vi "View.vi"(8 "error in (no error)":errorcluster, 11 "Thermal Chamber Controller In":refnum<class "Thermal Chamber Controller.lvclass">) -> (0 "error out":errorcluster)   [LabVIEW 2020, in "Thermal Chamber Controller.lvclass"]
doc: "This VI implements the main UI of the process. A reference to this VI should be set using the Set View VI Reference.vi method when the VI is started."
uses:
  Thermal Chamber Controller.lvclass
  C:/Program Files (x86)/National Instruments/LabVIEW 2020/vi.lib/Astemes/Triarc Framework/Process/Process.lvclass
  C:/Program Files (x86)/National Instruments/LabVIEW 2020/vi.lib/Astemes/Triarc Framework/View/View.lvclass
  <vilib>/Astemes/Triarc Framework/View/View.lvclass/View.ctl
  Thermal Chamber Controller.lvclass/Thermal Chamber Controller.ctl
  Private/Heater State.ctl
  <vilib>/Astemes/Triarc Framework/View/View.lvclass
  <vilib>/Astemes/Triarc Framework/Process/Process.lvclass
  C:/Program Files (x86)/National Instruments/LabVIEW 2020/vi.lib/Asteme/Triarc Framework/View/View.lvclass
  C:/Program Files (x86)/National Instruments/LabVIEW 2020/vi.lib/Asteme/Triarc Framework/Process/Process.lvclass
  C:/Program Files (x86)/National Instruments/LabVIEW 2020/vi.lib/Asteme/Triarc Framework/Base/Base.lvclass
  C:/Program Files (x86)/National Instruments/LabVIEW 2020/vi.lib/Asteme/Triarc Framework/Error Handler Interface/Error Handler Interface.lvclass
  C:/Program Files (x86)/National Instruments/LabVIEW 2020/vi.lib/Asteme/Triarc Framework/Logging/Logging.lvclass
  C:/Users/anton/Documents/GitHub/Triarc-Examples/Thermal Chamber/Thermal Chamber Controller/Thermal Chamber Controller.lvclass
  C:/Program Files (x86)/National Instruments/LabVIEW 2020/vi.lib/Asteme/Triarc Framework/Helper Loop/Helper Loop.lvclass
panel:
  in  "Enable Heater":bool
  in  "Disable Heater":bool
  in  "Ramp Rate (deg C / second)":dbl=1.0
  in  "Temperature Set Point (deg C)":dbl=22.0
  out "Heater State":bool
  out "Actual Temperature":dbl format="%.2f"
  out "Chamber Temperature Chart":T1(graph)
  out "Status":string
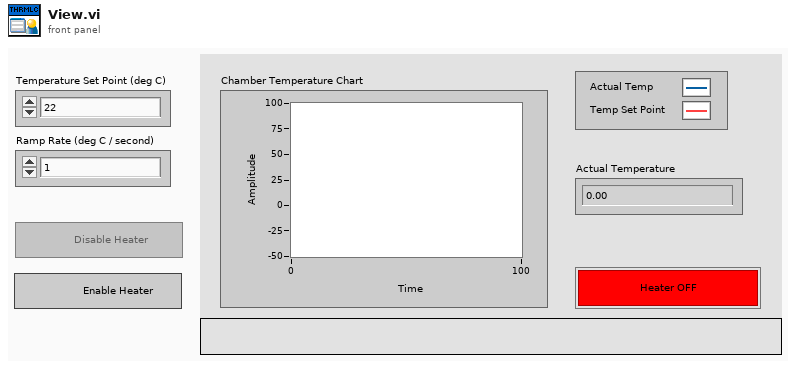
[diagram p1: front panel]
types:
  T1 = cluster{"Actual Temperature":dbl, "Required Temperature deg C":dbl}
  T2 = cluster{"Actual Temperature":dbl, "Required Temperature deg C":dbl}[]
  T3 = typedef "Thermal Chamber Controller.lvclass/Heater State.ctl" = enum16{"Heater Disabled", "Heater Enabled"}
  T4 = cluster{"Actual Temperature":dbl, "Temperature Set Point":dbl}
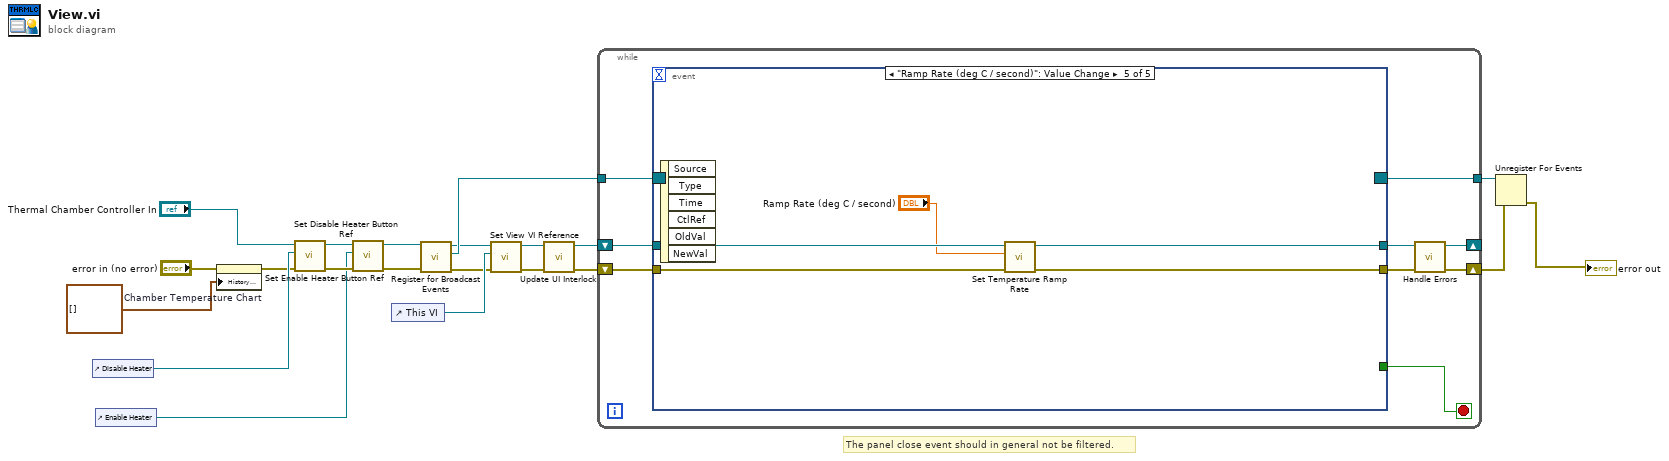
[diagram p0: block diagram]
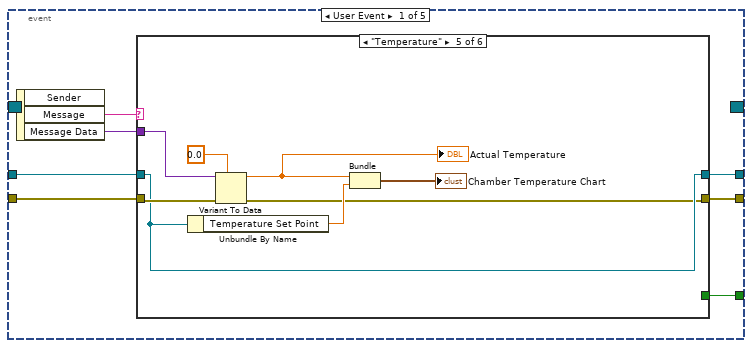
[diagram p2: hidden frame]
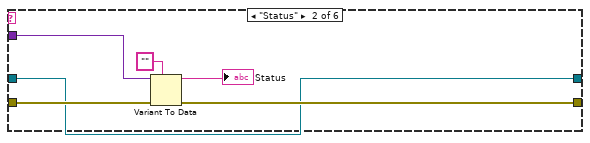
[diagram p4: hidden frame]
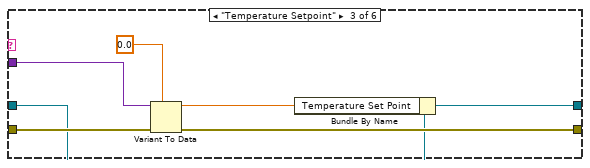
[diagram p5: hidden frame]
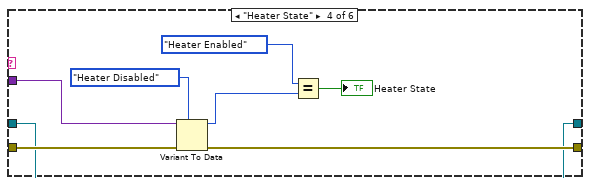
[diagram p6: hidden frame]
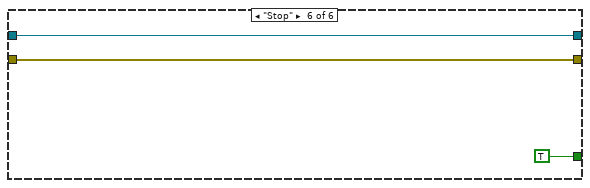
[diagram p7: hidden frame]
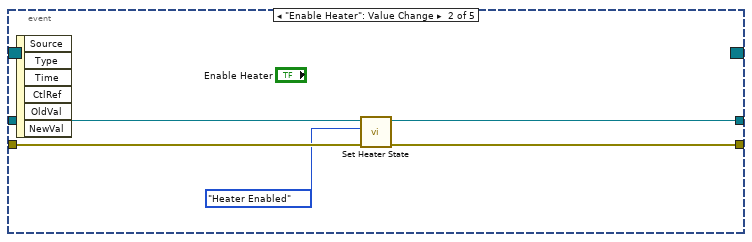
[diagram p8: hidden frame]
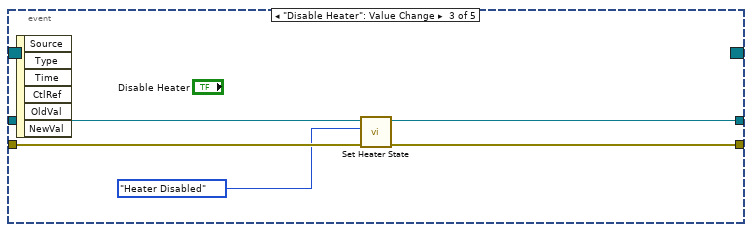
[diagram p9: hidden frame]
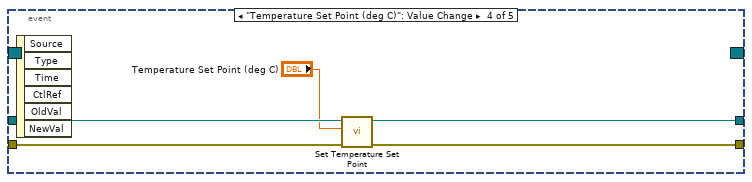
[diagram p10: hidden frame]
diagram:
  # "The panel close event should in general not be filtered."
  n1 = control-ref of="Disable Heater"() -> (w8:refnum<vi>)
  n2 = control-ref of="Enable Heater"() -> (w7:refnum<vi>)
  n3 = property on="Chamber Temperature Chart" class="WFChart (strict)"(error in="error in (no error)", "History Data"=T2 []) -> (error out=w2:errorcluster)  [unwired: 1 in, 1 out]
  n4 = call "Set Disable Heater Button Ref.vi"("error in (no error)"=w2, "Disable Heater Button Ref"=w8, "Thermal Chamber Controller In"="Thermal Chamber Controller In") -> ("error out"=w11:errorcluster, "Thermal Chamber Controller Out"=w9:refnum<class "Thermal Chamber Controller.lvclass">)  [unwired: 7 in]
  n5 = call "Set Enable Heater Button Ref.vi"("error in (no error)"=w11, "Enable Heater Button Ref"=w7, "Thermal Chamber Controller In"=w9) -> ("error out"=w13:errorcluster, "Thermal Chamber Controller Out"=w12:refnum<class "Thermal Chamber Controller.lvclass">)  [unwired: 7 in]
  n6 = control-ref of="This VI"() -> (w20:refnum<vi>)
  n7 = call <vilib>:"Register for Broadcast Events.vi"("error in (no error)"=w13, "Process In"=w12) -> ("error out"=w18:errorcluster, "Event Registration Refnum Out"=w19:refnum<event-registration>, "Process Out"=w17:refnum<class "Thermal Chamber Controller.lvclass">)  [unwired: 7 in]
  n8 = call <vilib>:"Set View VI Reference.vi"("error in (no error)"=w18, "View VI Reference"=w20, "View In"=w17) -> ("error out"=w16:errorcluster, "View Out"=w5:refnum<class "Thermal Chamber Controller.lvclass">)  [unwired: 7 in]
  n9 = call "Update UI Interlock.vi"("error in (no error)"=w16, "Thermal Chamber Controller In"=w5) -> ("error out"=w6:errorcluster, "Thermal Chamber Controller Out"=w4:refnum<class "Thermal Chamber Controller.lvclass">)  [unwired: 8 in]
  n10 = while {
    shift-right: [w24] -> _
    shift-left: w4 -> [w30]
    shift-right: [w22] -> w15
    shift-left: w6 -> [w28]
    tunnel: w19 -> [w27]
    tunnel: [w26] -> w14
    stop <- w25 stop-if-true
    n11 = event shown="[4] \"Ramp Rate (deg C / second)\": Value Change" {
      selector: w27 -> [_ _ _ _ _]
      dyn-events: [_ _ _ _ _] -> w26
      timeout: _ -> [_ _ _ _ _]
      tunnel: w30 -> [w37 w74 w79 w86 w89]
      tunnel: [w36 w73 w78 w85 w88] -> w29
      tunnel: w28 -> [w34 w76 w81 w83 w91]
      tunnel: [w35 w75 w80 w84 w90] -> w23
      tunnel: [w32 _ _ _ _] -> w25
      event User Event {
        n12 = event-data() -> ("Message"=w33:string, "Message Data"=w31:variant)  [unwired: 1 in, 1 out]
        n13 = case shown="\"Temperature\"" w33 {
          tunnel: w37 -> [w39 w40 w49 w53 w63 w71]
          tunnel: [w39 w40 w47 w53 w63 w71] -> w36
          tunnel: [w38 w41 w50 w57 w62 w70] -> w35
          tunnel: w34 -> [w38 w44 w51 w58 w68 w70]
          tunnel: [_ _ _ _ _ TRUE] -> w32
          tunnel: w31 -> [_ w45 w52 w59 w67 _]
          frame Default {
          }
          frame "Status" {
            n14 = Variant To Data(error in=w44, type="", Variant=w45) -> (data=→"Status":string, error out=w41:errorcluster)
          }
          frame "Temperature Setpoint" {
            n15 = Variant To Data(error in=w51, type=0.0 ("Numeric"), Variant=w52) -> (data=w46:dbl, error out=w50:errorcluster)
            n16 = Bundle By Name(cluster=w49, "Temperature Set Point"=w46) -> (w47:refnum<class "Thermal Chamber Controller.lvclass">)
          }
          frame "Heater State" {
            n17 = Variant To Data(error in=w58, type=Heater_State."Heater Disabled" ("Heater State"), Variant=w59) -> (data=w55:T3, error out=w57:errorcluster)
            n18 = Equal?(x=Heater_State."Heater Enabled" ("Heater State"), y=w55) -> (x = y?=→"Heater State":bool)
          }
          frame "Temperature" {
            n19 = Unbundle By Name(w63) -> ("Temperature Set Point"=w64:dbl)
            n20 = Variant To Data(error in=w68, type=0.0 ("Actual Temperature"), Variant=w67) -> (data=w65:dbl, error out=w62:errorcluster)
            "Actual Temperature" <- w65
            n21 = Bundle("Actual Temperature"=w65, "Temperature Set Point"=w64) -> (→"Chamber Temperature Chart":T4)  [unwired: 1 in]
          }
          frame "Stop" {
          }
        }
      }
      event "Enable Heater": Value Change {
        n22 = event-data() -> ()  [unwired: 1 in, 6 out]
        n23 = call "Set Heater State.vi"("error in (no error)"=w76, "Heater State"=Heater_State."Heater Enabled", "Thermal Chamber Controller In"=w74) -> ("error out"=w75:errorcluster, "Thermal Chamber Controller Out"=w73:refnum<class "Thermal Chamber Controller.lvclass">)  [unwired: 7 in]
      }
      event "Disable Heater": Value Change {
        n24 = event-data() -> ()  [unwired: 1 in, 6 out]
        n25 = call "Set Heater State.vi"("error in (no error)"=w81, "Heater State"=Heater_State."Heater Disabled", "Thermal Chamber Controller In"=w79) -> ("error out"=w80:errorcluster, "Thermal Chamber Controller Out"=w78:refnum<class "Thermal Chamber Controller.lvclass">)  [unwired: 7 in]
      }
      event "Temperature Set Point (deg C)": Value Change {
        n26 = event-data() -> ()  [unwired: 1 in, 6 out]
        n27 = call "Set Temperature Set Point.vi"("error in (no error)"=w83, "Temperature Set Point"="Temperature Set Point (deg C)", "Thermal Chamber Controller In"=w86) -> ("error out"=w84:errorcluster, "Thermal Chamber Controller Out"=w85:refnum<class "Thermal Chamber Controller.lvclass">)  [unwired: 7 in]
      }
      event "Ramp Rate (deg C / second)": Value Change {
        n28 = event-data() -> ()  [unwired: 1 in, 6 out]
        n29 = call "Set Temperature Ramp Rate.vi"("error in (no error)"=w91, "Temperature Ramp Rate [degC/s]"="Ramp Rate (deg C / second)", "Thermal Chamber Controller In"=w89) -> ("error out"=w90:errorcluster, "Thermal Chamber Controller Out"=w88:refnum<class "Thermal Chamber Controller.lvclass">)  [unwired: 7 in]
      }
    }
    n30 = call-dynamic "Handle Errors.vi"("error in (no error)"=w23, "Process In"=w29) -> ("error out"=w22:errorcluster, "Process Out"=w24:refnum<class "Thermal Chamber Controller.lvclass">)  [unwired: 8 in]
  }
  n31 = Unregister For Events(event registration refnum=w14, error in=w15) -> (error out=→"error out":errorcluster)
